vi "TestAirmar.vi"() -> ()   [LabVIEW 2013]
uses:
  Data/TypeDefs/AirmarStatus.ctl
  Data/TypeDefs/UTM Location.ctl
  <vilib>/myRIO/Common/Instrument Driver Framework/myRIO v1.0/UART/vis/myRIO v1.0 Close UART.vi
  <vilib>/myRIO/Common/Instrument Driver Framework/Utilities/vis/FPGA Ref Manager.vi
  <vilib>/myRIO/Common/Instrument Driver Framework/myRIO v1.0/myRIO v1.0 Reset FPGA.vi
  <vilib>/myRIO/Instrument Drivers/Utilities/Utilities.lvlib
panel:
  out "VISA read buffer":string
  out "Stop  Button\nHeartbeat":bool
  out "Stop Button\nLoop modulo":i32
  out "Total number of connection attempts":i32
  out "Loop modulo":i32
  out "Heartbeat":bool
  out "Wind Speed":dbl
  out "Wind Direction":dbl
  out "Roll":dbl
  out "Pitch":dbl
  out "Boat Speed":dbl
  out "Boat Direction":dbl
  out "Boat Location":T1 {"North" format="%#_10f"; "East" format="%#_8f"}
  out "Airmar Status":T2={"Sensor Connected"=TRUE, "Sensor Initialized"=TRUE, "Sensor OK"=TRUE, "Latest Error String"=TRUE, "GPS Lock"=FALSE}
  in  "stop":bool
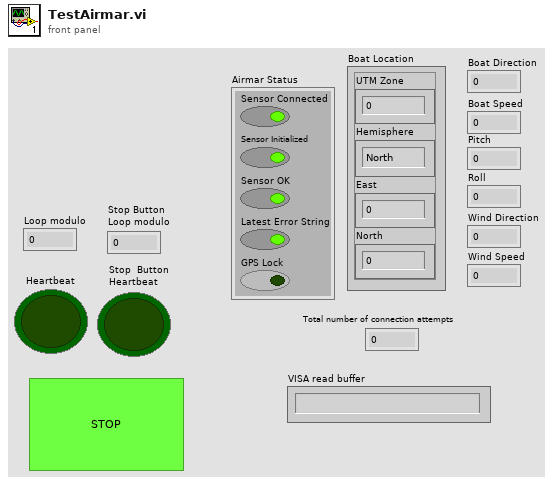
[diagram p1: front panel]
types:
  T1 = typedef "UTM Location.ctl" = cluster{"UTM Zone":dbl, "Hemisphere":enum16{"North", "South"}, "East":dbl, "North":dbl}
  T2 = typedef "AirmarStatus.ctl" = cluster{"Sensor Connected":bool, "Sensor Initialized":bool, "Sensor OK":bool, "Latest Error String":bool, "GPS Lock":bool}
  T3 = typedef "Notifiers.ctl" = cluster{"BoatSpeed":refnum<notifier>, "WindSpeed":refnum<notifier>, "MissionCheckOff":refnum<notifier>, "EStop":refnum<notifier>, "SpeedOverWater":refnum<notifier>, "BoatDirection":refnum<notifier>, "Luffing":refnum<notifier>, "RudderForce":refnum<notifier>, "BatteryVoltage":refnum<notifier>, "StayForces":refnum<notifier>, "BoatLocation":refnum<notifier>, "Pitch":refnum<notifier>, "Roll":refnum<notifier>, "RateOfTurn":refnum<notifier>, "RelWindDirection":refnum<notifier>, "SailPositions":refnum<notifier>, "RudderPosition":refnum<notifier>, "IronsRange":refnum<notifier>, "AbsWindDirection":refnum<notifier>, "OverrideInformation":refnum<notifier>, "DynamixelTorques":refnum<notifier>, "HardwareOnline?":refnum<notifier>, "MotorSetup":refnum<notifier>, "Airmar Status":refnum<notifier>, "BoatType":refnum<notifier>}
  T4 = typedef "WindData Queue Cluster.ctl" = cluster{"RelWindDirection Queue":refnum<queue>, "WindSpeed Queue":refnum<queue>, "AbsWindDirection Queue":refnum<queue>}
  T5 = typedef "GPS-Compass Queue Cluster.ctl" = cluster{"BoatLocation Queue":refnum<queue>, "BoatDirection Queue":refnum<queue>, "BoatSpeed Queue":refnum<queue>, "RateOfTurn Queue":refnum<queue>, "Pitch Queue":refnum<queue>, "Roll Queue":refnum<queue>}
  T6 = typedef "Sail Set Suggestions.ctl" = cluster{"MainSailSuggestion":dbl, "JibSailSuggestion":dbl}
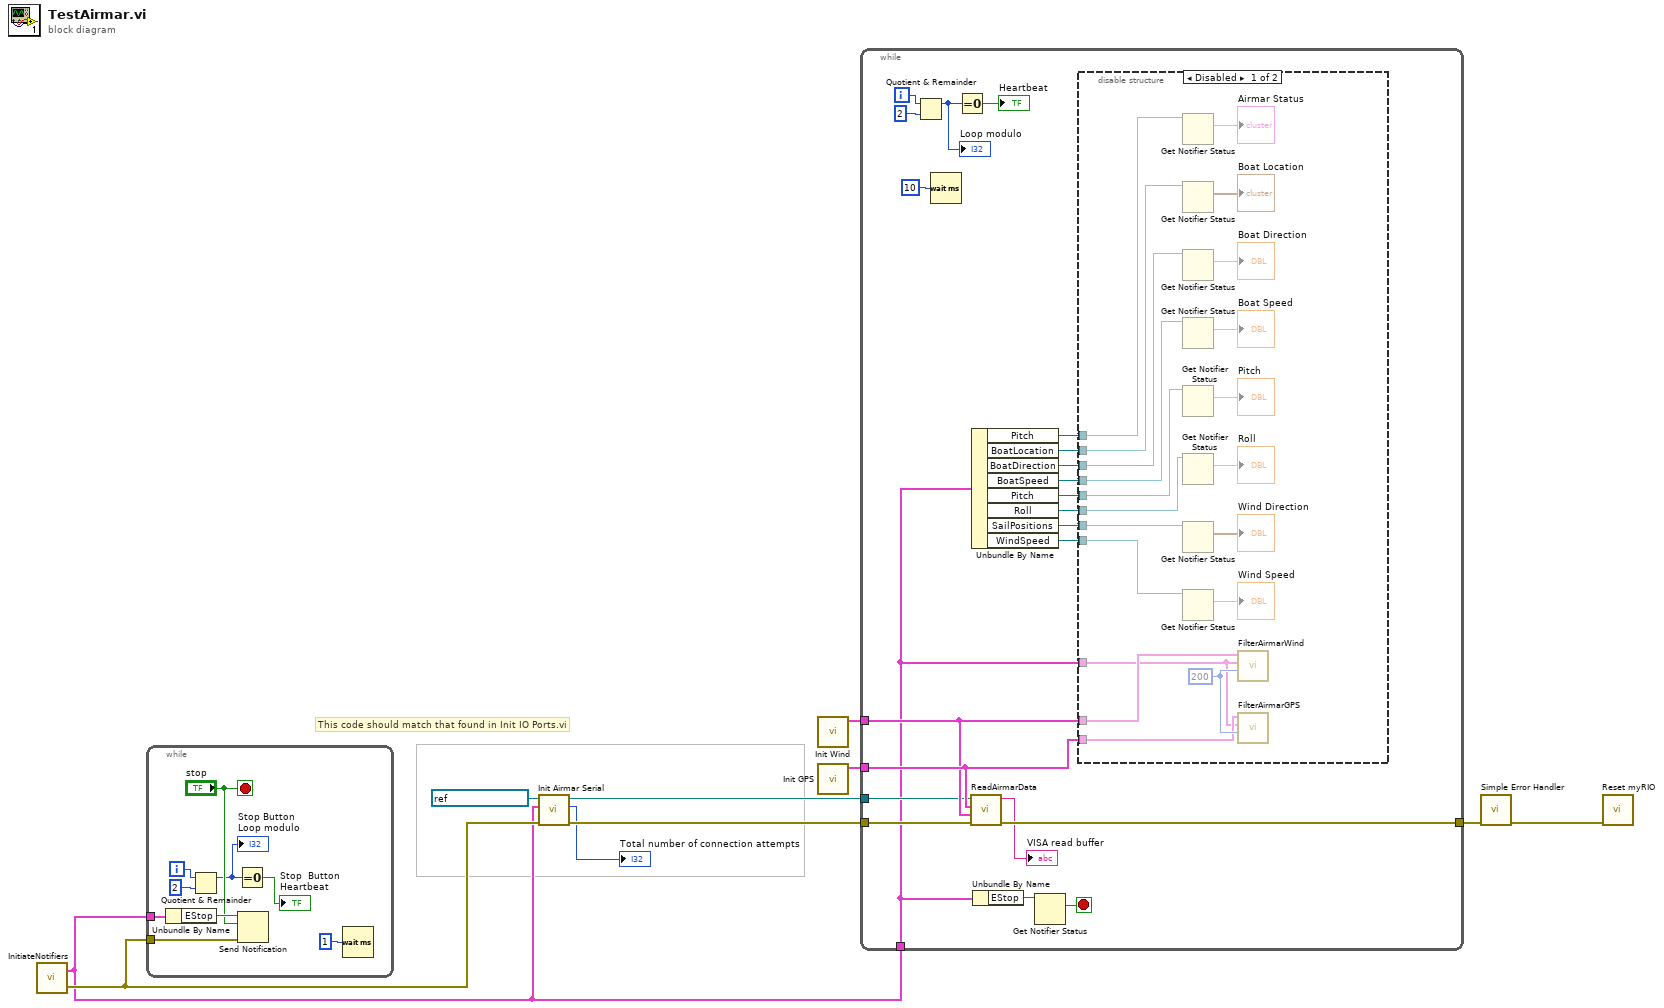
[diagram p0: block diagram]
diagram:
  # "This code should match that found in Init IO Ports.vi"
  n1 = call "InitiateNotifiers.vi"() -> ("error out"=w2:errorcluster, "NotifierReferences"=w1:T3)  [unwired: 2 in]
  n2 = while {
    tunnel: w1 -> [w17]
    tunnel: w2 -> [w11]
    i -> [w13]
    stop <- "stop" stop-if-true
    n3 = Unbundle By Name(w17) -> ("EStop"=w18:refnum<notifier>)
    n4 = Quotient & Remainder(x=w13, y=2) -> (x-y*floor(x/y)=w12:i32)  [unwired: 1 out]
    "Stop Button\nLoop modulo" <- w12
    n5 = Equal To 0?(x=w12) -> (x = 0?=→"Stop  Button\nHeartbeat":bool)
    n6 = Send Notification(notification="stop", notifier=w18, error in (no error)=w11) -> ()  [unwired: 2 out]
    n7 = Wait (ms)(milliseconds to wait=u32 1) -> ()  [unwired: 1 out]
  }
  n8 = call "Init Airmar Serial.vi"("error in (no error)"=w2, "NotifierReff"=w1, "VISA Refnum in"=refnum<visa-resource-name> "ASRL1::INSTR") -> ("error out"=w5:errorcluster, "Total number of connection attempts"=→"Total number of connection attempts":i32, "VISA Refnum out"=w6:refnum<visa-resource-name>)  [unwired: 6 in]
  n9 = call "Init Wind.vi"() -> ("Wind Queue Cluster"=w10:T4)  [unwired: 11 in]
  n10 = call "Init GPS.vi"() -> ("GPS-Compass Queue Cluster"=w9:T5)  [unwired: 11 in]
  n11 = while {
    tunnel: w10 -> [w39]
    tunnel: w9 -> [w40]
    tunnel: w1 -> [w23]
    tunnel: [w27] -> w8
    tunnel: w6 -> [w25]
    tunnel: w5 -> [w24]
    i -> [w30]
    stop <- w21 stop-if-true
    n12 = Quotient & Remainder(x=w30, y=2) -> (x-y*floor(x/y)=w26:i32)  [unwired: 1 out]
    "Loop modulo" <- w26
    n13 = Wait (ms)(milliseconds to wait=u32 10) -> ()  [unwired: 1 out]
    n14 = Equal To 0?(x=w26) -> (x = 0?=→"Heartbeat":bool)
    n15 = call "ReadAirmarData.vi"("Error in"=w24, "Airmar Wind Queue Cluster"=w39, "AirmarGPS-Compass Queue Cluster"=w40, "VISA UART port"=w25) -> ("Error out"=w27:errorcluster, "VISA read buffer"=→"VISA read buffer":string)  [unwired: 6 in]
    n16 = Unbundle By Name(w23) -> ("Pitch"=w38:refnum<notifier>, "BoatLocation"=w37:refnum<notifier>, "BoatDirection"=w36:refnum<notifier>, "BoatSpeed"=w35:refnum<notifier>, "Pitch"=w34:refnum<notifier>, "Roll"=w33:refnum<notifier>, "SailPositions"=w32:refnum<notifier>, "WindSpeed"=w31:refnum<notifier>)
    n17 = Unbundle By Name(w23) -> ("EStop"=w22:refnum<notifier>)
    n18 = Get Notifier Status(notifier=w22) -> (current notification=w21:bool)  [unwired: 1 in, 4 out]
    n19 = disable-structure shown="Disabled" {
      disable-tunnel: w40 -> [w60 _]
      disable-tunnel: w39 -> [w59 _]
      disable-tunnel: w23 -> [w58 _]
      disable-tunnel: w38 -> [w57 _]
      disable-tunnel: w37 -> [w56 _]
      disable-tunnel: w36 -> [w55 _]
      disable-tunnel: w35 -> [w54 _]
      disable-tunnel: w34 -> [w53 _]
      disable-tunnel: w33 -> [w52 _]
      disable-tunnel: w32 -> [w51 _]
      disable-tunnel: w31 -> [w50 _]
      frame Disabled {
        w61 = 200 ("Queue timeout (ms)")
        n20 = Get Notifier Status(notifier=w57) -> (current notification=→"Airmar Status":dbl)  [unwired: 1 in, 4 out]
        n21 = Get Notifier Status(notifier=w56) -> (current notification=→"Boat Location":T1)  [unwired: 1 in, 4 out]
        n22 = Get Notifier Status(notifier=w55) -> (current notification=→"Boat Direction":dbl)  [unwired: 1 in, 4 out]
        n23 = Get Notifier Status(notifier=w54) -> (current notification=→"Boat Speed":dbl)  [unwired: 1 in, 4 out]
        n24 = Get Notifier Status(notifier=w53) -> (current notification=→"Pitch":dbl)  [unwired: 1 in, 4 out]
        n25 = Get Notifier Status(notifier=w52) -> (current notification=→"Roll":dbl)  [unwired: 1 in, 4 out]
        n26 = Get Notifier Status(notifier=w51) -> (current notification=→"Wind Direction":T6)  [unwired: 1 in, 4 out]
        n27 = Get Notifier Status(notifier=w50) -> (current notification=→"Wind Speed":dbl)  [unwired: 1 in, 4 out]
        n28 = call "FilterAirmarWind.vi"("Queue timeout (ms)"=w61, "NotifierReff"=w58, "Airmar Wind Queue Cluster"=w59) -> ()  [unwired: 9 in]
        n29 = call "FilterAirmarGPS.vi"("Queue timeout (ms)"=w61, "NotifierReff"=w58, "AirmarGPS-Compass Queue Cluster"=w60) -> ()  [unwired: 9 in]
      }
      frame Enabled {
      }
    }
  }
  n30 = call <vilib>:"Simple Error Handler.vi"("error in (no error)"=w8) -> ("error out"=w7:errorcluster)  [unwired: 4 in, 4 out]
  n31 = call <vilib>:"Reset myRIO.vi"("error in (no error)"=w7) -> ()  [unwired: 10 in, 1 out]
